vi "Boolean Operator.vi"() -> ()   [LabVIEW 2019]
panel:
  in  "Boolean 2":bool
  in  "Boolean":bool
  out ".not. (x .or. y)?":bool
  out ".not. (x .and. y)?":bool
  out "x .or. y?":bool
  out "x .and. y?":bool
  # "Align the Indicators Properly"
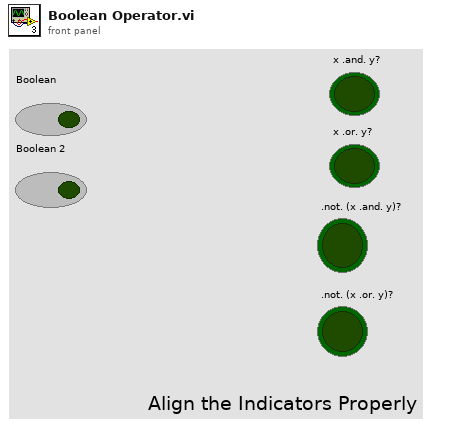
[diagram p1: front panel]
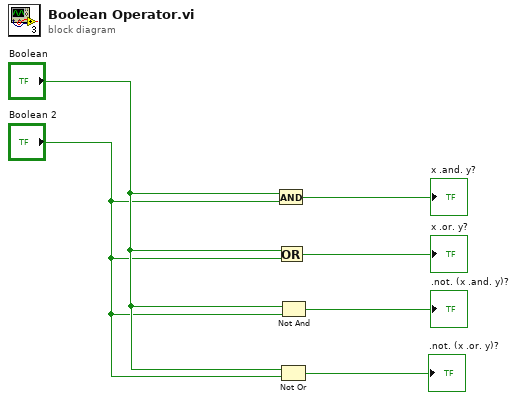
[diagram p0: block diagram]
diagram:
  n1 = And(x="Boolean", y="Boolean 2") -> (x .and. y?=→"x .and. y?":bool)
  n2 = Or(x="Boolean", y="Boolean 2") -> (x .or. y?=→"x .or. y?":bool)
  n3 = Not Or(1:"Boolean 2", 2:"Boolean") -> (0:→".not. (x .or. y)?":bool)
  n4 = Not And(1:"Boolean 2", 2:"Boolean") -> (0:→".not. (x .and. y)?":bool)
